vi "MIC_416_Subvi-identifier_noev3.vi"(11 "BrickReference in":T1) -> (2 "Array":dbl[](array[numeric]), 3 "BrickReference out":T1)   [LabVIEW 2016]
uses:
  <vilib>/NXT/Block Support/NXT_InputPort.ctl
  <vilib>/NXT/Dual Mode Library/prims/inRangeAndCoerce/inRangeAndCoerce_int.vi
  <vilib>/NXT/Dual Mode Library/Sensors/EV3_Color_RGB.vi
  <vilib>/NXT/Dual Mode Library/Sensors/Touch_Pressed.vi
  <vilib>/NXT/Dual Mode Library/Sensors/EV3_Color_Color.vi
  <vilib>/NXT/LegoClasses/BrickReference/BrickReference.lvclass
  <vilib>/NXT/Subs/LVHSConnector.ctl
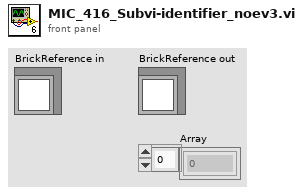
[diagram p1: front panel]
types:
  T1 = typedef "LVHSConnector.ctl" = refnum<class "BrickReference.lvclass">
  T2 = typedef "NXT_InputPort.ctl" = u32
  T3 = typedef "ColorSensorColors.ctl" = enum16{"No Color", "Black", "Blue", "Green", "Yellow", "Red", "White", "Brown"}
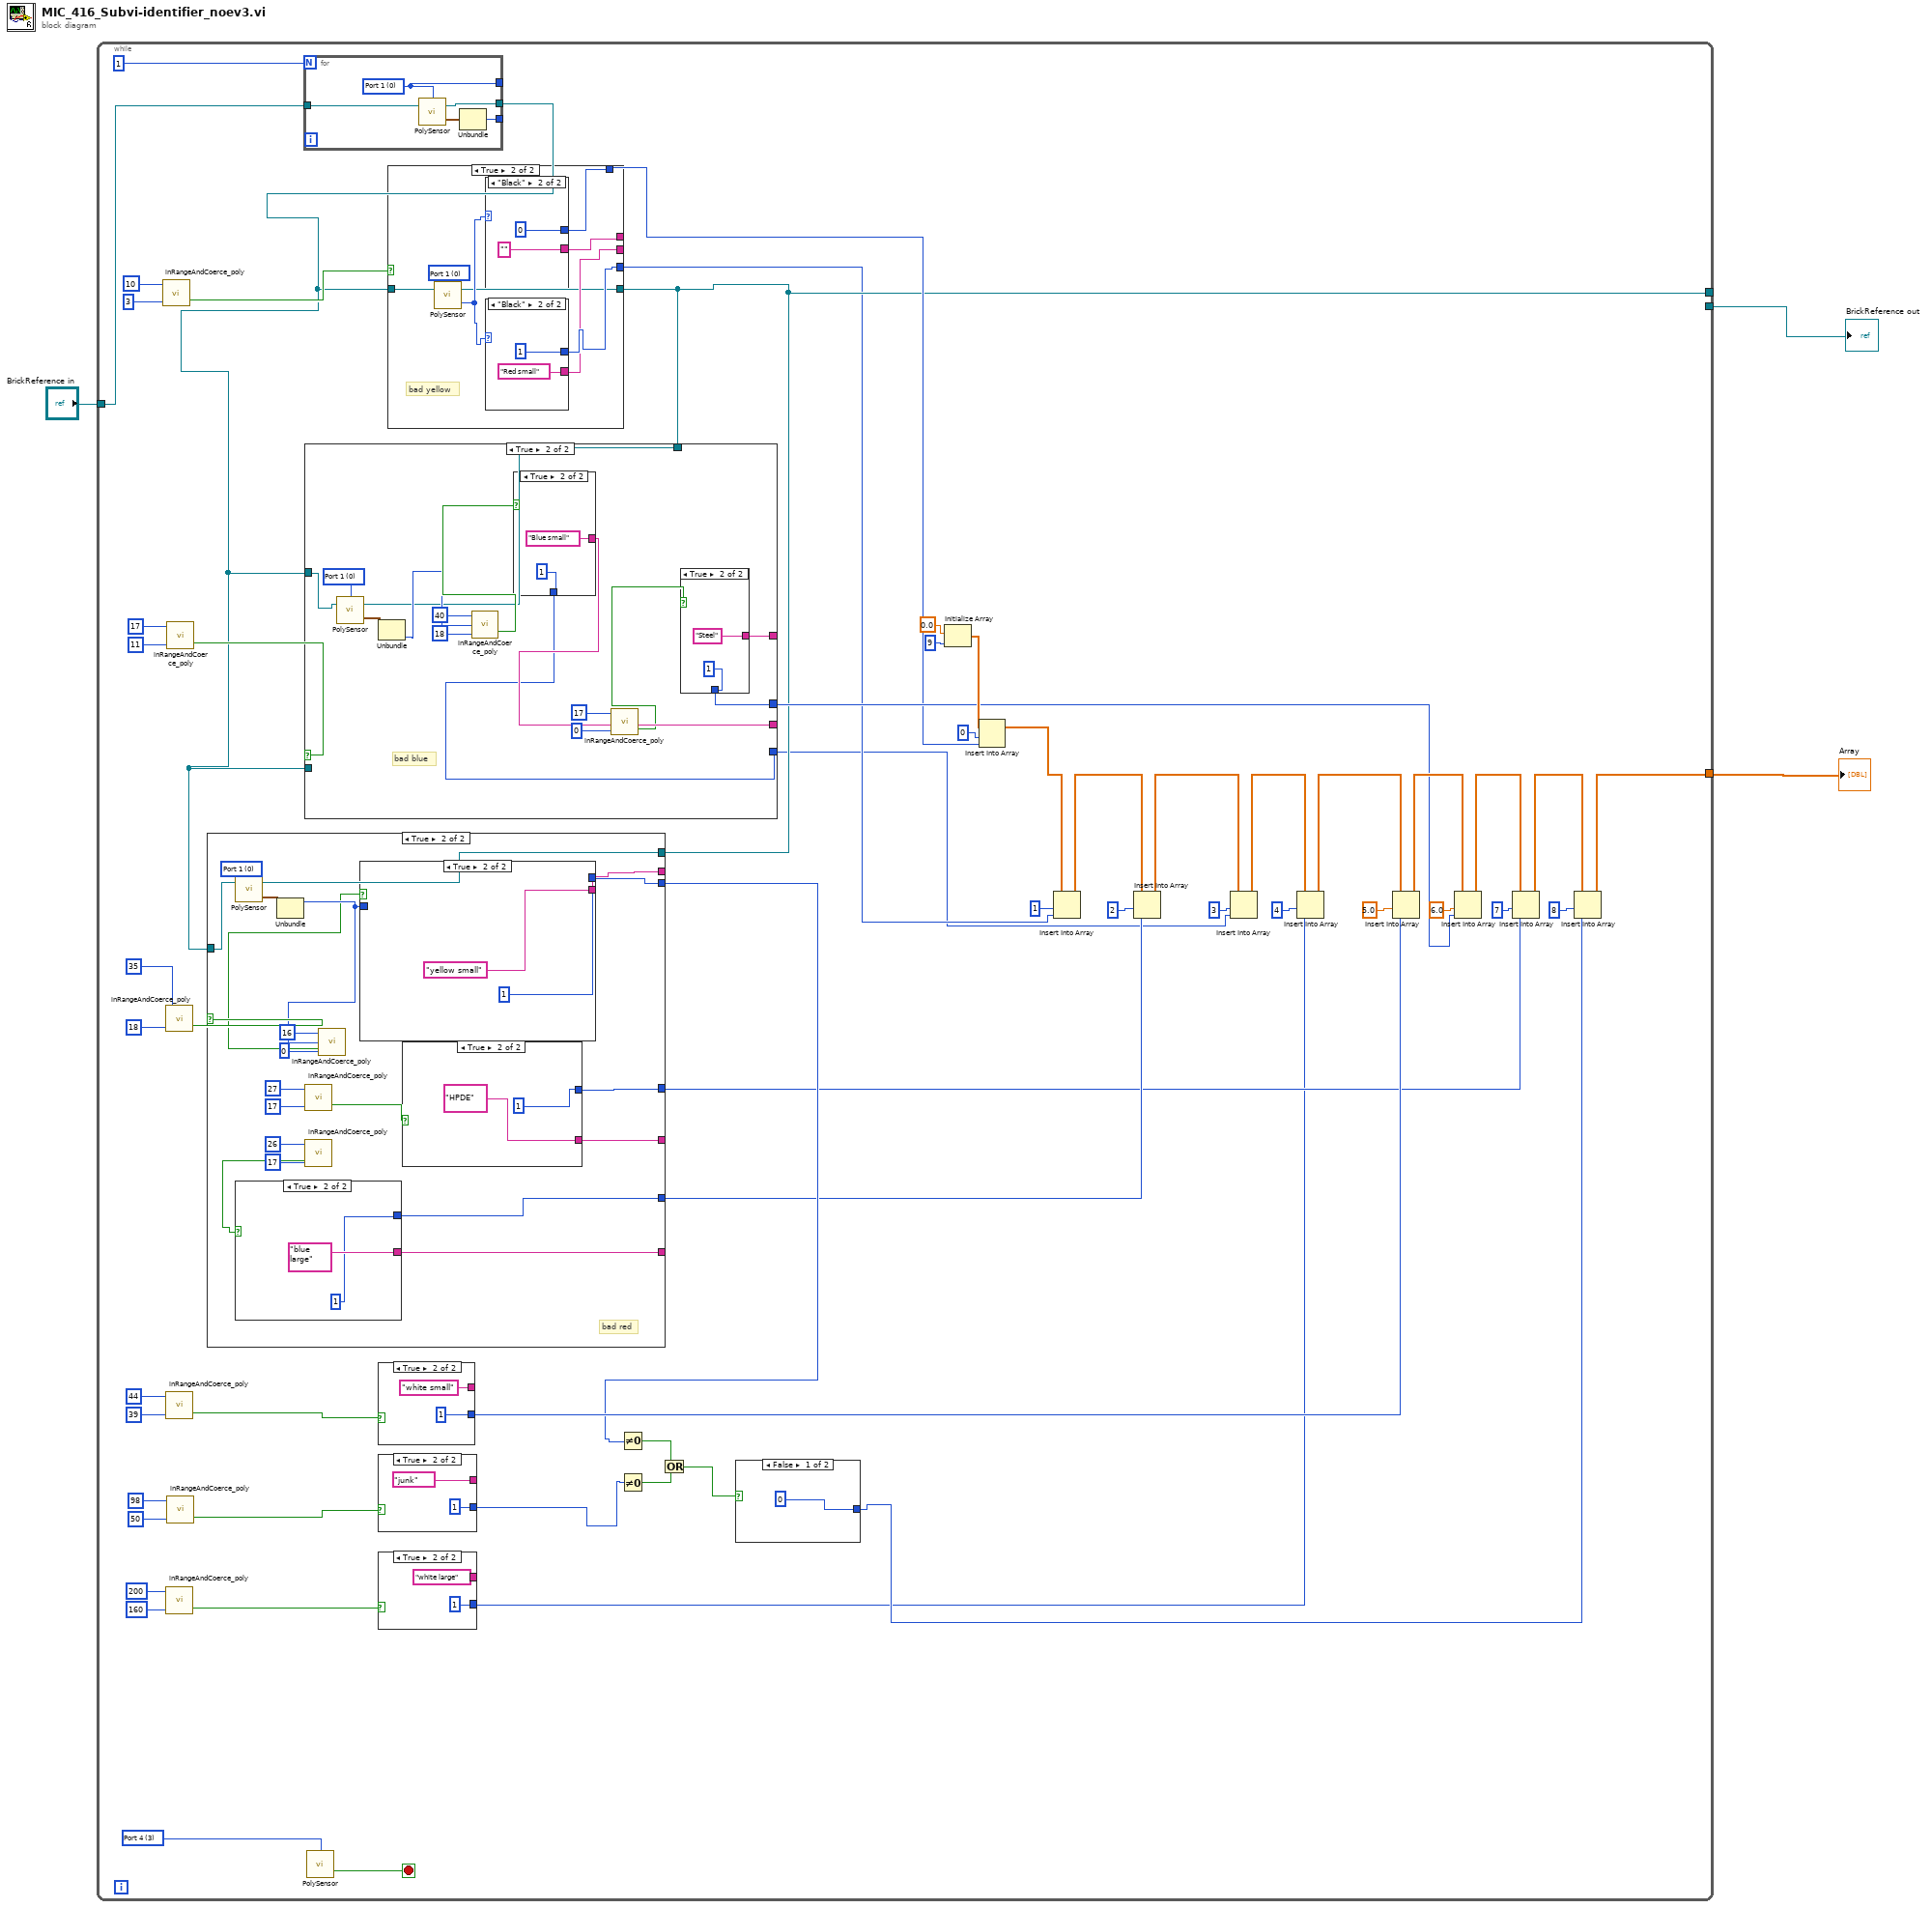
[diagram p0: block diagram]
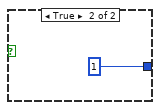
[diagram p2: hidden frame]
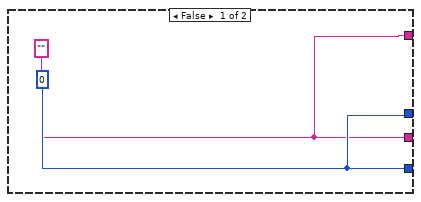
[diagram p3: hidden frame]
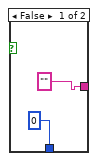
[diagram p4: hidden frame]
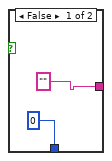
[diagram p5: hidden frame]
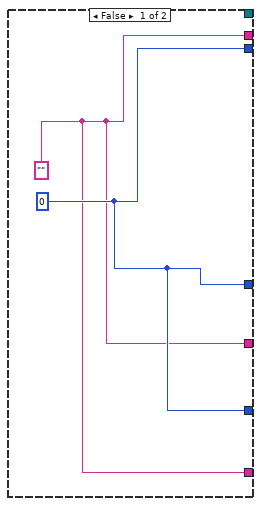
[diagram p6: hidden frame]
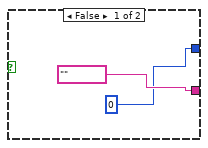
[diagram p7: hidden frame]
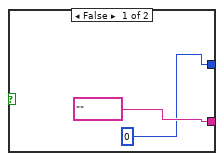
[diagram p8: hidden frame]
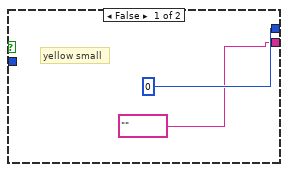
[diagram p9: hidden frame]
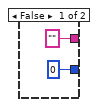
[diagram p10: hidden frame]
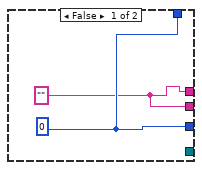
[diagram p11: hidden frame]
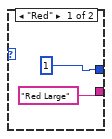
[diagram p12: hidden frame]
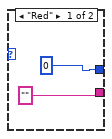
[diagram p13: hidden frame]
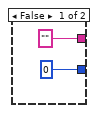
[diagram p14: hidden frame]
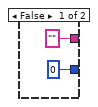
[diagram p15: hidden frame]
diagram:
  n1 = while {
    tunnel: "BrickReference in" -> [w20]
    tunnel: [w39] -> w2
    tunnel: [_] -> w3
    tunnel: [w7] -> _
    stop <- w61 stop-if-true
    w60 = T2 3 items=["Port 1", "Port 2", "Port 3", "Port 4"] ("Port (Port 1)")
    n2 = call-poly <vilib>:"inRangeAndCoerce_poly.vi"("lower limit"=3, "upper limit"=10) -> ("In Range?"=w30:bool)  [unwired: 1 in, 1 out]
    n3 = call-poly <vilib>:"inRangeAndCoerce_poly.vi"("lower limit"=18, "upper limit"=35) -> ("In Range?"=w24:bool)  [unwired: 1 in, 1 out]
    n4 = call-poly <vilib>:"inRangeAndCoerce_poly.vi"("lower limit"=39, "upper limit"=44) -> ("In Range?"=w33:bool)  [unwired: 1 in, 1 out]
    n5 = call-poly <vilib>:"inRangeAndCoerce_poly.vi"("lower limit"=160, "upper limit"=200) -> ("In Range?"=w36:bool)  [unwired: 1 in, 1 out]
    n6 = call-poly <vilib>:"inRangeAndCoerce_poly.vi"("lower limit"=11, "upper limit"=17) -> ("In Range?"=w21:bool)  [unwired: 1 in, 1 out]
    n7 = call-poly <vilib>:"inRangeAndCoerce_poly.vi"("lower limit"=50, "upper limit"=98) -> ("In Range?"=w27:bool)  [unwired: 1 in, 1 out]
    n8 = for {
      N: 1 -> [_]
      tunnel: w20 -> [w157]
      tunnel: [w156] -> _
      tunnel: [w155] -> w19
      tunnel: [w154] -> _
      w154 = T2 0 items=["Port 1", "Port 2", "Port 3", "Port 4"] ("Port (Port 1)")
      n9 = call-poly <vilib>:"PolySensor.vi"("NXT/EV3"=w157, "Port (Port 1)"=w154) -> ("RGB Color"=w158:cluster{"Red":u8, "Green":u8, "Blue":u8}, "NXT/EV3"=w155:T1)  [unwired: 1 in]
      n10 = Unbundle(w158) -> ("Green"=w156:u8)  [unwired: 2 out]
    }
    n11 = call-poly <vilib>:"PolySensor.vi"("Port (Port 1)"=w60) -> ("Yes / No"=w61:bool)  [unwired: 2 in, 1 out]
    n12 = case shown="True" w33 {
      tunnel: ["" "white small"] -> _
      tunnel: [0 1] -> w18
      frame False {
      }
      frame True {
      }
    }
    n13 = case shown="True" w27 {
      tunnel: ["" "junk"] -> _
      tunnel: [0 1] -> w15
      frame False {
      }
      frame True {
      }
    }
    n14 = case shown="True" w36 {
      tunnel: ["" "white large"] -> _
      tunnel: [0 1] -> w4
      frame False {
      }
      frame True {
      }
    }
    n15 = case shown="True" w30 {
      tunnel: [w129 w134] -> w6
      tunnel: w19 -> [_ w136]
      tunnel: [w129 w130] -> _
      tunnel: [w128 w133] -> _
      tunnel: [w128 w132] -> _
      tunnel: [_ w131] -> w7
      tunnel: [_ w130] -> w8
      frame False {
        w129 = 0
        w128 = ""
      }
      frame True {
        w137 = T2 0 items=["Port 1", "Port 2", "Port 3", "Port 4"] ("Port (Port 1)")
        # "bad yellow"
        n16 = call-poly <vilib>:"PolySensor.vi"("NXT/EV3"=w136, "Port (Port 1)"=w137) -> ("Detected Color"=w135:T3, "NXT/EV3"=w131:T1)  [unwired: 1 in]
        n17 = case shown="\"Black\"" w135 {
          tunnel: ["Red Large" ""] -> w132
          tunnel: [1 0] -> w130
          frame "Red" {
          }
          frame "Black" {
          }
        }
        n18 = case shown="\"Black\"" w135 {
          tunnel: ["" "Red small"] -> w133
          tunnel: [0 1] -> w134
          frame "Red" {
          }
          frame "Black" {
          }
        }
      }
    }
    n19 = case shown="True" w24 {
      tunnel: [w90 w106] -> _
      tunnel: [w91 w105] -> w12
      tunnel: [w91 w104] -> w11
      tunnel: [w91 w103] -> w10
      tunnel: [w90 w95] -> _
      tunnel: [w90 w94] -> _
      tunnel: w19 -> [_ w93]
      tunnel: w7 -> [_ w92]
      frame False {
        w91 = 0
        w90 = ""
      }
      frame True {
        w110 = T2 0 items=["Port 1", "Port 2", "Port 3", "Port 4"] ("Port (Port 1)")
        # "bad red"
        n20 = call-poly <vilib>:"PolySensor.vi"("NXT/EV3"=w93, "Port (Port 1)"=w110) -> ("RGB Color"=w111:cluster{"Red":u8, "Green":u8, "Blue":u8}, "NXT/EV3"=w92:T1)  [unwired: 1 in]
        n21 = Unbundle(w111) -> ("Red"=w107:u8)  [unwired: 2 out]
        n22 = call-poly <vilib>:"inRangeAndCoerce_poly.vi"("lower limit"=17, "upper limit"=27) -> ("In Range?"=w96:bool)  [unwired: 1 in, 1 out]
        n23 = call-poly <vilib>:"inRangeAndCoerce_poly.vi"("lower limit"=17, "upper limit"=26) -> ("In Range?"=w97:bool)  [unwired: 1 in, 1 out]
        n24 = case shown="True" w97 {
          tunnel: ["" "blue large"] -> w94
          tunnel: [0 1] -> w104
          frame False {
          }
          frame True {
          }
        }
        n25 = call-poly <vilib>:"inRangeAndCoerce_poly.vi"("lower limit"=0, "x"=w107, "upper limit"=16) -> ("In Range?"=w98:bool)  [unwired: 1 out]
        n26 = case shown="True" w98 {
          tunnel: ["" "yellow small"] -> w106
          tunnel: w107 -> [_ _]
          tunnel: [0 1] -> w105
          frame False {
            # "yellow small"
          }
          frame True {
          }
        }
        n27 = case shown="True" w96 {
          tunnel: ["" "HPDE"] -> w95
          tunnel: [0 1] -> w103
          frame False {
          }
          frame True {
          }
        }
      }
    }
    n28 = case shown="True" w21 {
      tunnel: [w65 w76] -> _
      tunnel: [w66 w74] -> w5
      tunnel: w19 -> [_ _]
      tunnel: [w66 w70] -> w9
      tunnel: [w65 w69] -> _
      tunnel: w19 -> [_ w68]
      tunnel: w7 -> [_ w67]
      frame False {
        w66 = 0
        w65 = ""
      }
      frame True {
        w80 = T2 0 items=["Port 1", "Port 2", "Port 3", "Port 4"] ("Port (Port 1)")
        # "bad blue"
        n29 = call-poly <vilib>:"PolySensor.vi"("NXT/EV3"=w68, "Port (Port 1)"=w80) -> ("RGB Color"=w81:cluster{"Red":u8, "Green":u8, "Blue":u8}, "NXT/EV3"=w67:T1)  [unwired: 1 in]
        n30 = Unbundle(w81) -> ("Blue"=w75:u8)  [unwired: 2 out]
        n31 = call-poly <vilib>:"inRangeAndCoerce_poly.vi"("lower limit"=18, "x"=w75, "upper limit"=40) -> ("In Range?"=w77:bool)  [unwired: 1 out]
        n32 = case shown="True" w77 {
          tunnel: ["" "Blue small"] -> w76
          tunnel: [0 1] -> w74
          frame False {
          }
          frame True {
          }
        }
        n33 = call-poly <vilib>:"inRangeAndCoerce_poly.vi"("lower limit"=0, "upper limit"=17) -> ("In Range?"=w71:bool)  [unwired: 1 in, 1 out]
        n34 = case shown="True" w71 {
          tunnel: ["" "Steel"] -> w69
          tunnel: [0 1] -> w70
          frame False {
          }
          frame True {
          }
        }
      }
    }
    n35 = Not Equal To 0?(x=w12) -> (x != 0?=w17:bool)
    n36 = Not Equal To 0?(x=w15) -> (x != 0?=w16:bool)
    n37 = Or(x=w17, y=w16) -> (x .or. y?=w14:bool)
    n38 = case shown="False" w14 {
      tunnel: [0 1] -> w13
      frame False {
      }
      frame True {
      }
    }
    n39 = Initialize Array(0.0 ("element"), 9 ("dimension size")) -> (w53:dbl[])
    n40 = Insert Into Array(array=w53, index=0, new element=w8) -> (w52:dbl[])
    n41 = Insert Into Array(array=w52, index=1, new element=w6) -> (w51:dbl[])
    n42 = Insert Into Array(array=w51, index=2, new element=w11) -> (w50:dbl[])
    n43 = Insert Into Array(array=w50, index=3, new element=w5) -> (w49:dbl[])
    n44 = Insert Into Array(array=w49, index=4, new element=w4) -> (w42:dbl[])
    n45 = Insert Into Array(array=w42, index=5.0 ("new element/subarray"), new element=w18) -> (w48:dbl[])
    n46 = Insert Into Array(array=w48, index=6.0 ("new element/subarray"), new element=w9) -> (w47:dbl[])
    n47 = Insert Into Array(array=w47, index=7, new element=w10) -> (w46:dbl[])
    n48 = Insert Into Array(array=w46, index=8, new element=w13) -> (w39:dbl[])
  }
  "BrickReference out" <- w3
  "Array" <- w2
